vi "LV to ITX XY AutoPlot.vi"(4 "Wavenames":string[](array[string]), 6 "command string":string="Display 'y_#wave#' vs 'x_#wave#'\nAppendToGraph 'y_#wave#' vs 'x_#wave#'\nLabel bottom \"#labelX#\"\nLabel left \"#labelY#\"\nModifyGraph rgb('y_#wave#')=(#r#,#g#,#b#)\n\\\\s('y_#wave#') #label#\nModifyGraph mirror=1\nModifyGraph width=216\nModifyGraph height={Aspect,0.6}\nModifyGraph Log(bottom)=#bottomlog#\nModifyGraph Log(left)=#leftlog#", 7 "path":path=path "C:/Users/voodoo.SEAGATE/Desktop/datatest", 8 "error in":errorcluster, 9 "Notes":string, 10 "XY-Data []":cluster{"X  array":dbl[], "Y  Array":dbl[]}[](array[cluster]), 11 "LV to ITX":refnum<class "LV to ITX.lvclass">) -> (0 "error out":errorcluster, 2 "file":path=path "C:/Users/voodoo.SEAGATE/Desktop/datatest/datatest.000019.itx", 3 "LV to ITX out":refnum<class "LV to ITX.lvclass">)   [LabVIEW 2016, in "LV to ITX.lvclass"]
doc: "Write your XY data to ITX file. This AutoPlot VI adds commands to automatically create a graph in Igor to quickly view your data.\n\n-- path: base path to save data\n-- filename: base filename\n-- Notes: add any notes here to help you remember what experiment you did\n-- XY Array: Array of Clusters (ie, Array of XY graphs)\n-- wavenames: Give each data array a unique name such as \"time, bias, current,...\"\n-- X,Y Labels: For plotting in Igor. Can be ignored.\n-- X,Y Log: Do you wan to show X or Y on Log scale in Igor?"
uses:
  LV to ITX.lvclass
  Typedefs/Dictionary--cluster.ctl
  Typedefs/Filetype--enum.ctl
  LV to ITX.lvclass/LV to ITX.ctl
panel:
  in  "Data (Dictionary)":T1[](array[typedef])
  in  "X,Y Log":i32[](array[numeric])
  in  "X,Y Labels":string[](array[string])=["x label", "y label"]
  # "Below are relevant for creating graphs in Igor"
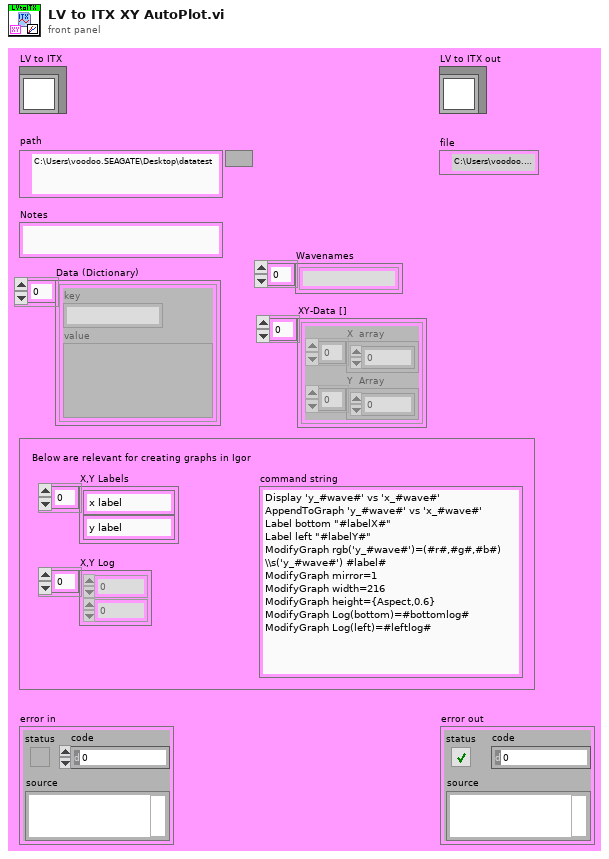
[diagram p1: front panel]
types:
  T1 = typedef "LV to ITX.lvclass/Dictionary--cluster.ctl" = cluster{"key":string, "value":variant}
  T2 = typedef "LV to ITX.lvclass/Filetype--enum.ctl" = enum16{"DAT", "ITX", "HDF5", "TDMS", "VI"}
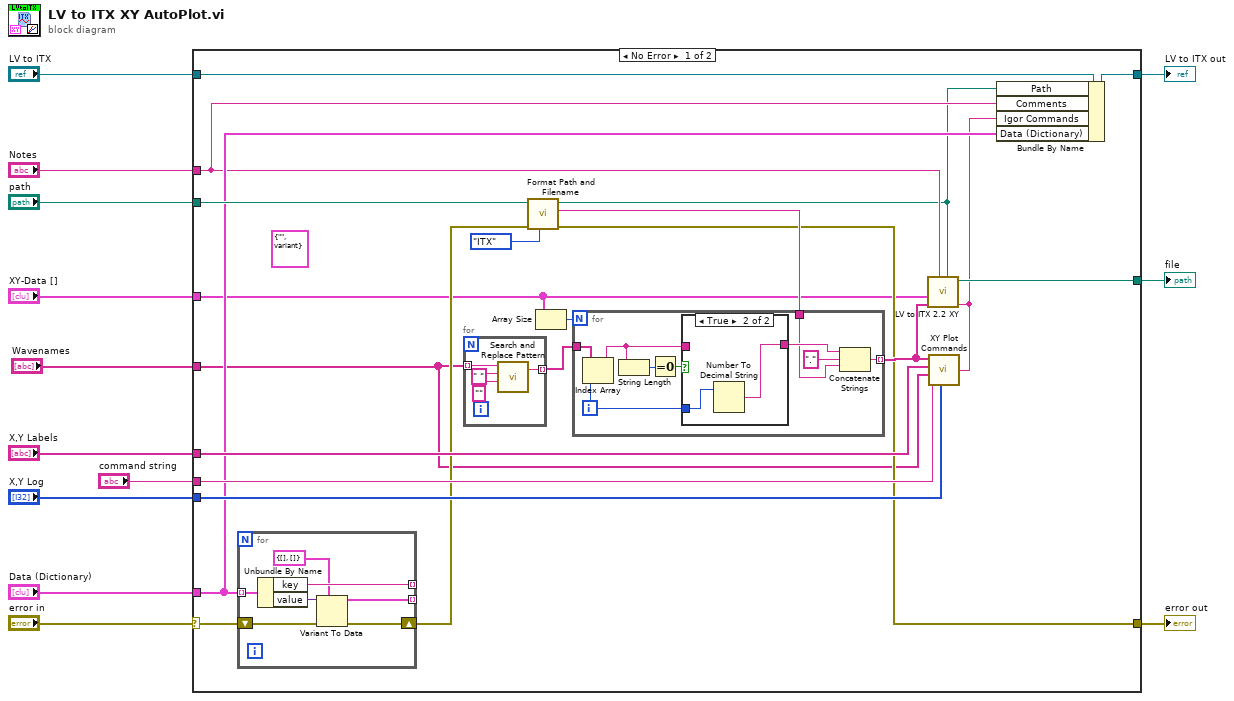
[diagram p0: block diagram]
diagram:
  n1 = case shown="No Error" "error in" {
    selector: "error in" -> [w20 w58]
    tunnel: "path" -> [w34 _]
    tunnel: "Notes" -> [w18 _]
    tunnel: "X,Y Labels" -> [w33 _]
    tunnel: [w32 _] -> w10
    tunnel: "X,Y Log" -> [w31 _]
    tunnel: "command string" -> [w26 _]
    tunnel: "Data (Dictionary)" -> [w19 _]
    tunnel: [w23 w58] -> w6
    tunnel: "LV to ITX" -> [w22 w59]
    tunnel: [w21 w59] -> w4
    tunnel: "XY-Data []" -> [w15 _]
    tunnel: "Wavenames" -> [w14 _]
    frame No Error {
      (unwired) T1 {"key"="", "value"=variant} ("key-value")
      n2 = for {
        tunnel: w19 -> [w41] mode=indexing
        shift-right: [w38] -> w24
        shift-left: w20 -> [w39]
        tunnel: [w37] -> _ mode=indexing
        tunnel: [w35] -> _ mode=indexing
        n3 = Unbundle By Name(w41) -> ("key"=w37:string, "value"=w40:variant)
        n4 = Variant To Data(error in=w39, type=cluster{"X  array":dbl[], "Y  Array":dbl[]} {"X  array"=[], "Y  Array"=[]} ("Averaged XY Graph"), Variant=w40) -> (data=w35:cluster{"X  array":dbl[], "Y  Array":dbl[]}, error out=w38:errorcluster)
      }
      n5 = for {
        tunnel: w14 -> [w57] mode=indexing
        tunnel: [w56] -> w30 mode=indexing
        n6 = call <vilib>:"Search and Replace Pattern.vi"("string"=w57, "regular expression (\"\")"=" " ("regular expression (\"\")"), "replace string (\"\")"="" ("replace string (\"\")")) -> ("result string"=w56:string)  [unwired: 2 in, 1 out]
      }
      n7 = call "Format Path and Filename.vi"("Type (TDMS)"=Filetype--enum."ITX", "error in"=w24, "path"=w34) -> ("error out"=w23:errorcluster, "filename without extension"=w28:string, "path"=w16:path)  [unwired: 6 in]
      n8 = Array Size(array=w15) -> (size(s)=w29:i32)
      n9 = for {
        N: w29 -> [_]
        tunnel: w30 -> [w45]
        tunnel: w28 -> [w42]
        tunnel: [w50] -> w27 mode=indexing
        i -> [w46]
        n10 = Index Array(array=w45, index=w46) -> (element=w44:string)
        n11 = String Length(string=w44) -> (length=w47:i32)
        n12 = Equal To 0?(x=w47) -> (x = 0?=w48:bool)
        n13 = case shown="True" w48 {
          tunnel: w46 -> [_ w52]
          tunnel: [w51 w53] -> w43
          tunnel: w44 -> [w51 _]
          frame False {
          }
          frame True {
            n14 = Number To Decimal String(number=w52) -> (decimal integer string=w53:string)  [unwired: 1 out]
          }
        }
        n15 = Concatenate Strings(w43, "." ("string"), w42) -> (w50:string)
      }
      n16 = call "XY Plot Commands.vi"("X,Y Log"=w31, "input string"=w26, "Plot labels"=w14, "X,Y Labels"=w33, "wavenames"=w27) -> ("result string"=w17:string)  [unwired: 1 in]
      n17 = call "LV to ITX 2.2 XY.vi"("Commands"=w17, "filename"=w16, "Notes"=w18, "wavenames"=w27, "XY Array"=w15) -> ("file"=w32:path)  [unwired: 6 in]
      n18 = Bundle By Name(cluster=w22, "Path"=w16, "Comments"=w18, "Igor Commands"=w17, "Data (Dictionary)"=w19) -> (w21:refnum<class "LV to ITX.lvclass">)
    }
    frame Error {
    }
  }
  "file" <- w10
  "error out" <- w6
  "LV to ITX out" <- w4
